vi "TweedieRegressor.vi"(8 "error in":errorcluster) -> (0 "error out":errorcluster, 3 "out":refnum<class "TweedieRegressor.lvclass">)   [LabVIEW 2020]
doc: "Generalized Linear Model with a Tweedie distribution.\n\n This estimator can be used to model different GLMs depending on the\n ``power`` parameter, which determines the underlying distribution.\n\n Read more in the :ref:`User Guide <Generalized_linear_regression>`.\n\n .. versionadded:: 0.23\n\n Parameters\n ----------\n power : float, default=0\n The power determines the underlying target distribution according\n to the following table:\n\n +-------+------------------------+\n | Power | Distribution |\n +=======+========================+\n | 0 | Normal |\n +-------+------------------------+\n | 1 | Poisson |\n +-------+------------------------+\n | (1,2) | Compound Poisson Gamma |\n +-------+------------------------+\n | 2 | Gamma |\n +-------+------------------------+\n | 3 | Inverse Gaussian |\n +-------+------------------------+\n\n For ``0 < power < 1``, no distribution exists.\n\n alpha : float, default=1\n Constant that multiplies the penalty term and thus determines the\n regularization strength. ``alpha = 0`` is equivalent to unpenalized\n GLMs. In this case, the design matrix `X` must have full column rank\n (no collinearities).\n\n fit_intercept : bool, default=True\n Specifies if a constant (a.k.a. bias or intercept) should be\n added to the linear predictor (X @ coef + intercept).\n\n link : {'auto', 'identity', 'log'}, default='auto'\n The link function of the GLM, i.e. mapping from linear predictor\n `X @ coeff + intercept` to prediction `y_pred`. Option 'auto' sets\n the link depending on the chosen family as follows:\n\n - 'identity' for Normal distribution\n - 'log' for Poisson, Gamma and Inverse Gaussian distributions\n\n max_iter : int, default=100\n The maximal number of iterations for the solver.\n\n tol : float, default=1e-4\n Stopping criterion. For the lbfgs solver,\n the iteration will stop when ``max{|g_j|, j = 1, ..., d} <= tol``\n where ``g_j`` is the j-th component of the gradient (derivative) of\n the objective function.\n\n warm_start : bool, default=False\n If set to ``True``, reuse the solution of the previous call to ``fit``\n as initialization for ``coef_`` and ``intercept_`` .\n\n verbose : int, default=0\n For the lbfgs solver set verbose to any positive number for verbosity.\n\n Attributes\n ----------\n coef_ : array of shape (n_features,)\n Estimated coefficients for the linear predictor (`X @ coef_ +\n intercept_`) in the GLM.\n\n intercept_ : float\n Intercept (a.k.a. bias) added to linear predictor.\n\n n_iter_ : int\n Actual number of iterations used in the solver.\n\n \nAvailable methods:\nGet Attributes\nGet Params\nSet Params"
uses:
  TweedieRegressor.lvclass
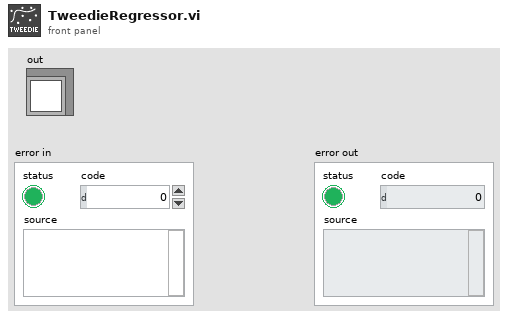
[diagram p1: front panel]
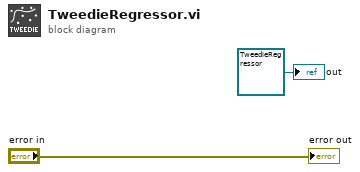
[diagram p0: block diagram]
diagram:
  "out" <- refnum<class "TweedieRegressor.lvclass"> refnum ("model")
  "error out" <- "error in"
